vi "performanceCalc2.vi"(0 "init":bool, 1 "windowLength":dbl, 3 "pckSuccess":dbl, 4 "pckTotal":dbl, 5 "delay":dbl, 6 "idx":dbl, 7 "errors":dbl[](array[numeric]), 10 "pckTotalTrack":dbl[](array[numeric]), 11 "prevPckTotal":dbl, 12 "prevErrors":dbl) -> (9 "currentError":dbl, 13 "prevPckTotalOut":dbl, 14 "currentIdx":dbl, 15 "errorsOut":dbl[](array[numeric]), 16 "pckTotalTrackOut":dbl[](array[numeric]), 17 "reliability":dbl format="%.2f", 18 "delayOut":dbl format="%.2f", 19 "prevErrorsOut":dbl)   [LabVIEW 2009]
uses:
  <vilib>/imath/engines/lvmath2/RunTimeEngine/BuiltInFunctions/mod/NIMS_mod_no_size_check.vi
  <vilib>/imath/engines/lvmath2/RunTimeEngine/ReplaceToken/NIMS_Replace - V(S)=S.vi
  <vilib>/imath/engines/lvmath2/RunTimeEngine/ReplaceToken/NIMS_Replace - Check(_) Linear.vi
  <vilib>/imath/engines/lvmath2/RunTimeEngine/ReplaceToken/NIMS_Replace - Size Check _(_)=S.vi
  <vilib>/imathl/engines/lvmath/Functions/Error Handling/Create Error.vi
  <vilib>/imath/engines/lvmath2/RunTimeEngine/VariableToken/Read/NIMS_Get Elements - RV(_) - Check(_).vi
  <vilib>/imath/engines/lvmath/Functions/Error Handling/MergeErrorsWrapper.vi
  <vilib>/imath/engines/lvmath2/RunTimeEngine/BuiltInFunctions/sum/NIMS_sum(GV).vi
  <vilib>/imath/engines/lvmath2/RunTimeEngine/NodeEndStatement/NIMS_NodeEndStatement_Output.vi
  <vilib>/imath/engines/lvmath2/RunTimeEngine/ErrorHandling/NIMS_Finalize Error.vi
  <vilib>/imath/engines/lvmath2/RunTimeEngine/Parser/MC_Version.vi
panel:
  in  "pckTotalTrack 2":dbl[](array[numeric])
  out "prevState":dbl[](array[numeric])
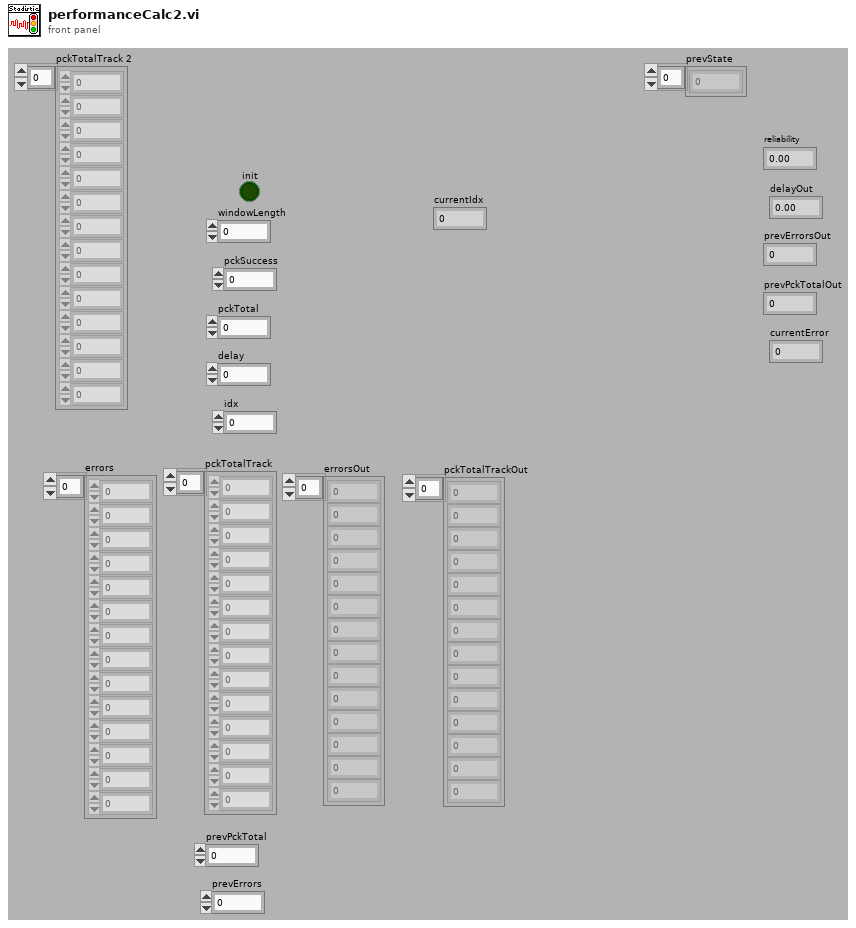
[diagram p1: front panel]
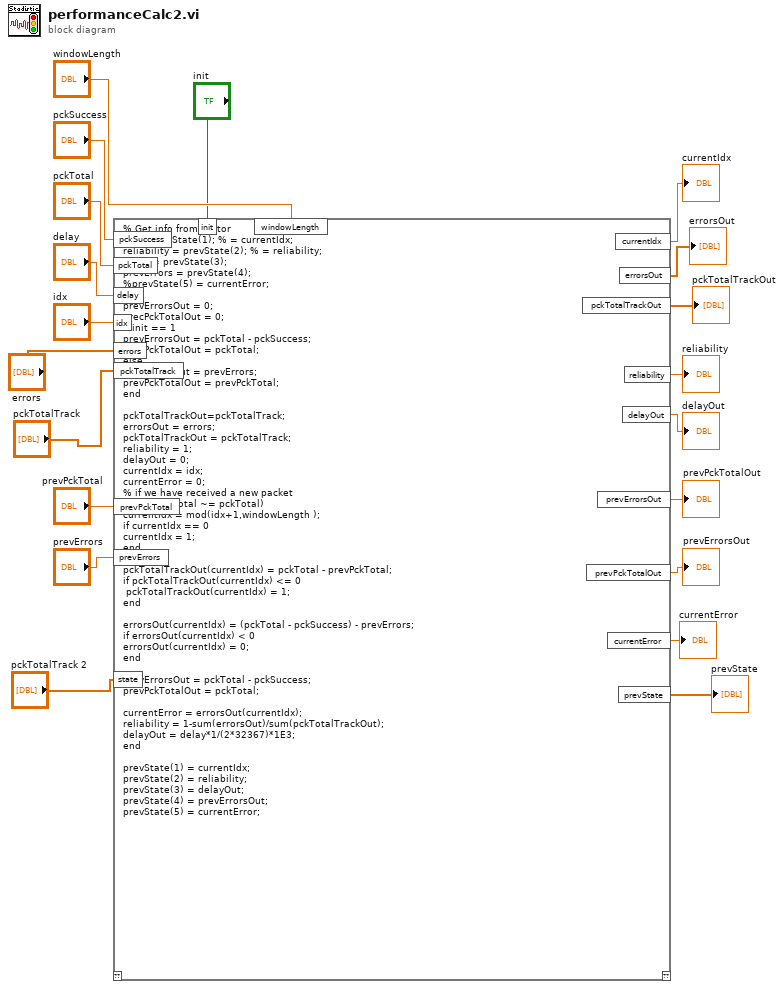
[diagram p0: block diagram]
diagram:
  n1 = mathscript code="% Get info from vector\nidx = prevState(1); % = currentIdx;\nreliability = prevState(2); % = reliability;\ndelay = prevState(3);\nprevErrors = prevState(4);\n%prevState(5) = currentError;\n\nprevErrorsOut = 0;\nprecPckTotalOut = 0;\nif init == 1\nprevErrorsOut = pckTotal - pckSuccess;\nprevPckTotalOut = pckTotal;\nelse\nprevErrorsOut = prevErrors;\nprevPckTotalOut = prevPckTotal;\nend\n\npckTotalTrackOut=pckTotalTrack;\nerrorsOut = errors;\npckTotalTrackOut = pckTotalTrack;\nreliability = 1;\ndelayOut = 0;\ncurrentIdx = idx;\ncurrentError = 0;\n% if we have received a new packet\nif (prevPckTotal ~= pckTotal)\ncurrentIdx = mod(idx+1,windowLength );\nif currentIdx == 0\ncurrentIdx = 1;\nend\n\npckTotalTrackOut(currentIdx) = pckTotal - prevPckTotal;\nif pckTotalTrackOut(currentIdx) <= 0\n pckTotalTrackOut(currentIdx) = 1;\nend\n\nerrorsOut(currentIdx) = (pckTotal - pckSuccess) - prevErrors;\nif errorsOut(currentIdx) < 0\nerrorsOut(currentIdx) = 0;\nend\n\nprevErrorsOut = pckTotal - pckSuccess;\nprevPckTotalOut = pckTotal;\n\ncurrentError = errorsOut(currentIdx);\nreliability = 1-sum(errorsOut)/sum(pckTotalTrackOut);\ndelayOut = delay*1/(2*32367)*1E3;\nend\n\nprevState(1) = currentIdx;\nprevState(2) = reliability;\nprevState(3) = delayOut;\nprevState(4) = prevErrorsOut;\nprevState(5) = currentError;"("pckSuccess"="pckSuccess", "pckTotal"="pckTotal", "delay"="delay", "idx"="idx", "errors"="errors", "pckTotalTrack"="pckTotalTrack", "windowLength"="windowLength", "prevPckTotal"="prevPckTotal", "prevErrors"="prevErrors", "init"="init", "state"="pckTotalTrack 2") -> ("currentIdx"=→"currentIdx":dbl, "errorsOut"=→"errorsOut":dbl[], "pckTotalTrackOut"=→"pckTotalTrackOut":dbl[], "reliability"=→"reliability":dbl, "delayOut"=→"delayOut":dbl, "prevErrorsOut"=→"prevPckTotalOut":dbl, "prevPckTotalOut"=→"prevErrorsOut":dbl, "currentError"=→"currentError":dbl, "prevState"=→"prevState":dbl[])  [unwired: 1 in, 1 out]
